vi "teleop3.vi"() -> ()   [LabVIEW 2012, in "Test.lvrbt"]
uses:
  Test.lvrbt
  <vilib>/NXT/Hardware/Plugins/Tetrix DC Motor/TetrixDCMotorAddress.ctl
  <vilib>/NXT/Block Support/NXT_OutputPort.ctl
  <vilib>/NXT/NXTIO Xnodes/NXTIONodeSubVIs/LEGOStopAllMotors.vi
  <vilib>/FTC/FTC Calculate Drive Power - Arcade Left.vi
  <vilib>/NXT/NXTIO Xnodes/NXTIONodeSubVIs/LEGOMoveAllMotors.vi
  <vilib>/FTC/FTC Interpret Motor Power From Right Y Axis.vi
  <vilib>/FTC/FTC Interpret Motor Power From Left Y Axis.vi
  <vilib>/NXT/NXTIO Xnodes/NXTIONodeSubVIs/TETRIX IO Move DC Motors.vi
  <vilib>/NXT/NXTIO Xnodes/NXTIONodeSubVIs/NXTMoveMotors.vi
  <vilib>/NXT/NXTIO Xnodes/NXTIONodeSubVIs/NXTStopMotors.vi
  <vilib>/NXT/NXTIO Xnodes/NXTIONodeSubVIs/TETRIX IO Stop DC Motors.vi
  <vilib>/NXT/NXTIO Xnodes/NXTIONodeSubVIs/TETRIX IO Check Battery.vi
  <vilib>/NXT/Hardware/Plugins/Open Port/OpenPortAddress.ctl
  <vilib>/NXT/Subs/LVHSConnector.ctl
  <vilib>/NXT/NXTIO Xnodes/NXTIOXNode/NXTIO.xnode
  <vilib>/NXT/NXTIO Xnodes/AddressXNode/NXTIOAddress.xnode
  <vilib>/NXT/LegoClasses/BrickReference/BrickReference.lvclass
panel:
  in  "Drive Power 3":i8=75 min=-100 max=100
  in  "Drive Power 2":i8=75 min=-100 max=100
  in  "Drive Power":i8=75 min=-100 max=100
  # "You may modify the code as needed for your robot. To test this program for an FTC match, open to the Remote Control Editor, select the \"Run Program\" tab, and choose \"Teleop\"."
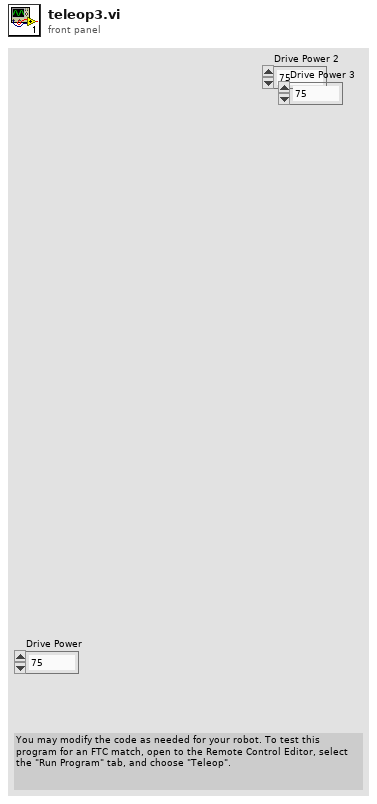
[diagram p1: front panel]
types:
  T1 = typedef "TetrixDCMotorAddress.ctl" = i32
  T2 = cluster{"TetrixDCMotor":T1, "TetrixDCMotor 2":T1}
  T3 = typedef "LVHSConnector.ctl" = refnum<class "BrickReference.lvclass">
  T4 = typedef "FTC ControllerState.ctl" = cluster{"Left X":i8, "Left Y":i8, "Right X":i8, "Right Y":i8, "Button Encoding 9-12":u8, "Button Encoding 1-8":u8, "POV":T5}
  T5 = typedef "FTC POVState.ctl" = i8
  T6 = typedef "FTC ButtonEventType.ctl" = enum16{"Pressed", "Released"}
  T7 = cluster{"Button ID":enum16{"None", "Button 1", "Button 2", "Button 3", "Button 4", "Button 5", "Button 6", "Button 7", "Button 8", "Button 9", "Button 10", "Button 11", "Button 12", "POV Up", "POV Up Right", "POV Right", "POV Down Right", "POV Down", "POV Down Left", "POV Left", "POV Up Left"}, "Event Type":T6}[]
  T8 = enum16{"None", "Button 1", "Button 2", "Button 3", "Button 4", "Button 5", "Button 6", "Button 7", "Button 8", "Button 9", "Button 10", "Button 11", "Button 12", "POV Up", "POV Up Right", "POV Right", "POV Down Right", "POV Down", "POV Down Left", "POV Left", "POV Up Left"}
  T9 = typedef "NXT_OutputPort.ctl" = u8
  T10 = typedef "FTC ButtonState.ctl" = cluster{"Button 1":bool, "Button 2":bool, "Button 3":bool, "Button 4":bool, "Button 5":bool, "Button 6":bool, "Button 7":bool, "Button 8":bool, "Button 9":bool, "Button 10":bool, "Button 11":bool, "Button 12":bool, "POV":T5}
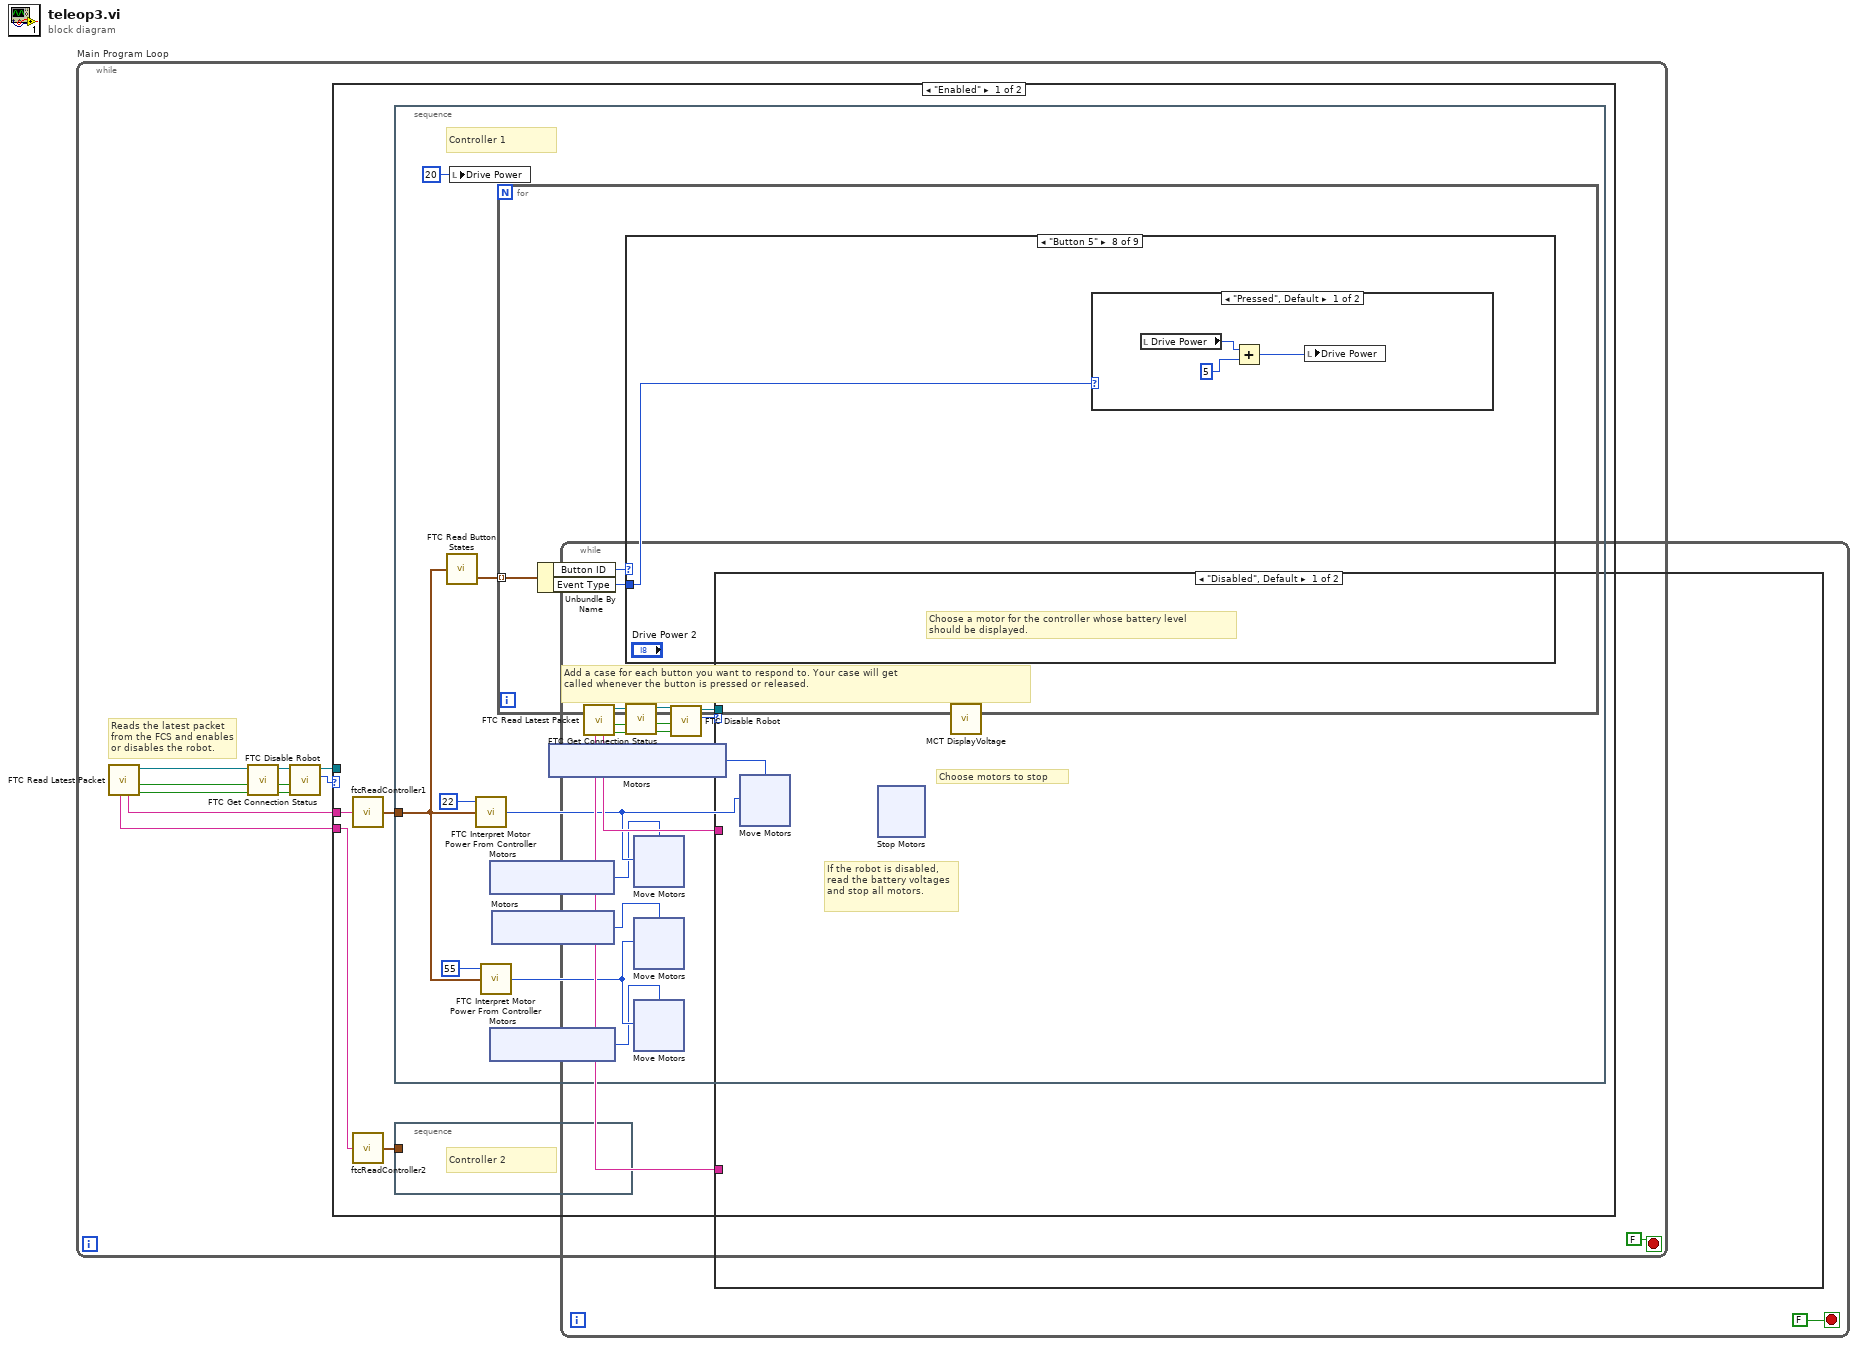
[diagram p0: block diagram]
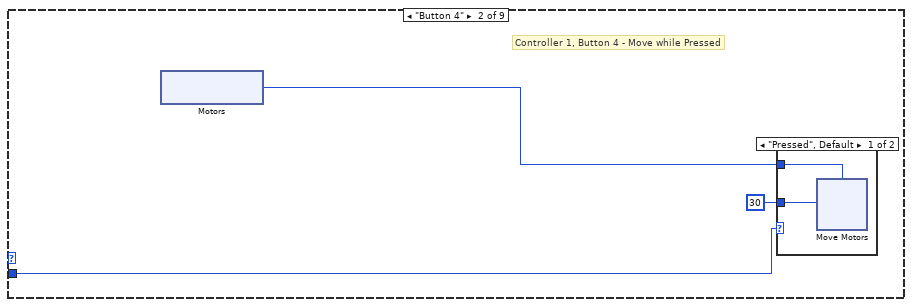
[diagram p3: hidden frame]
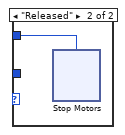
[diagram p4: hidden frame]
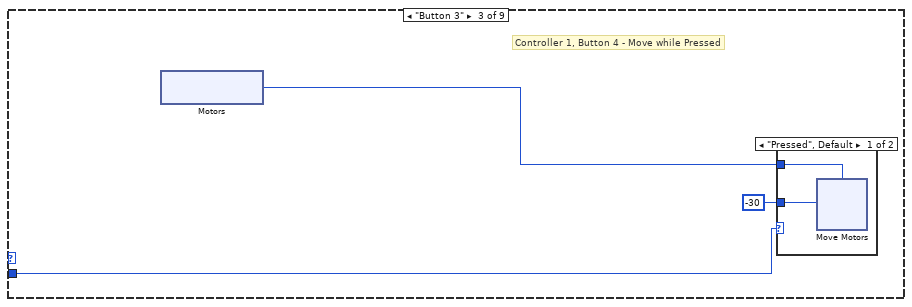
[diagram p5: hidden frame]
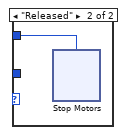
[diagram p6: hidden frame]
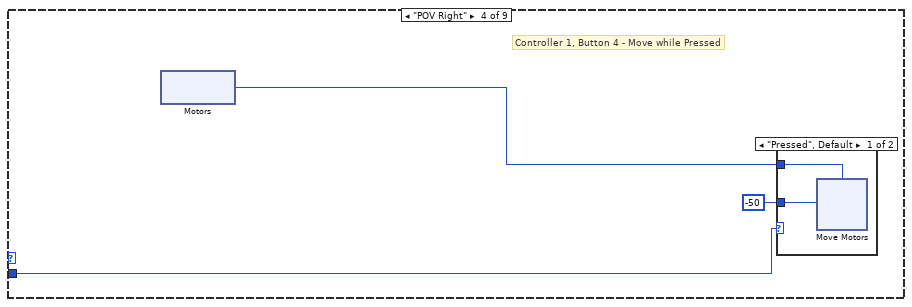
[diagram p7: hidden frame]
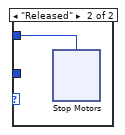
[diagram p8: hidden frame]
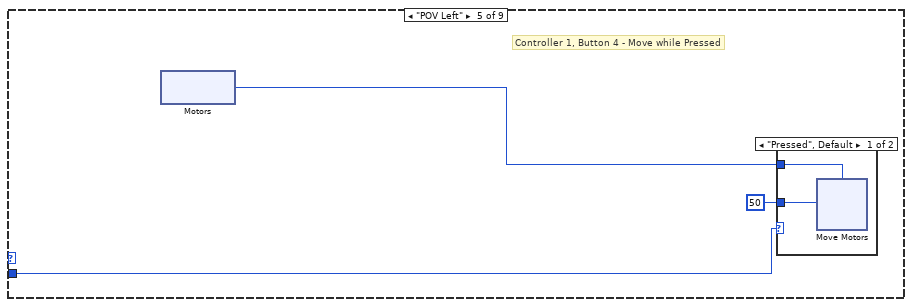
[diagram p9: hidden frame]
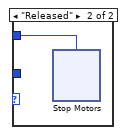
[diagram p10: hidden frame]
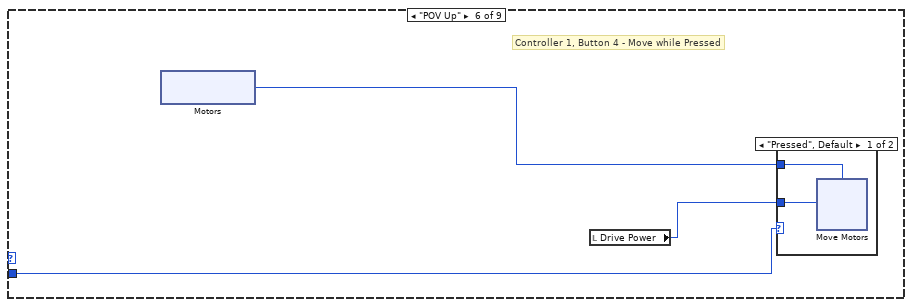
[diagram p11: hidden frame]
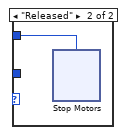
[diagram p12: hidden frame]
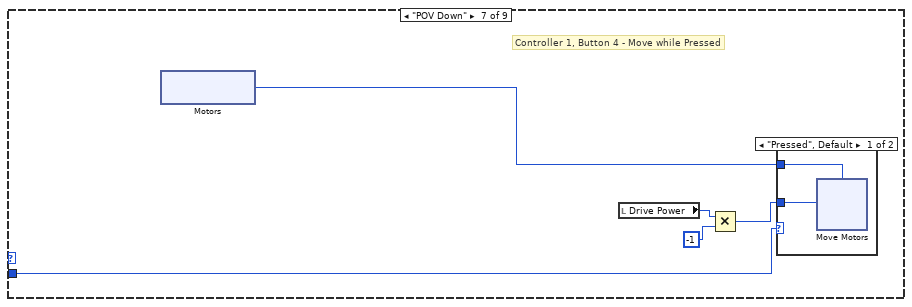
[diagram p13: hidden frame]
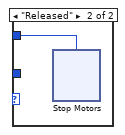
[diagram p14: hidden frame]
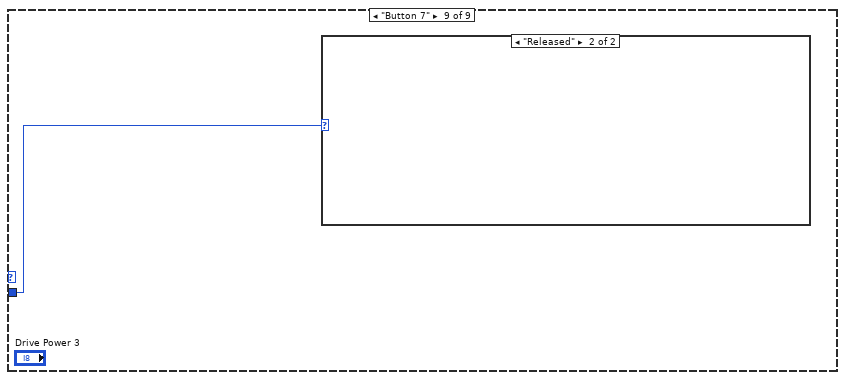
[diagram p16: hidden frame]
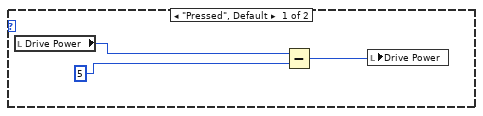
[diagram p17: hidden frame]
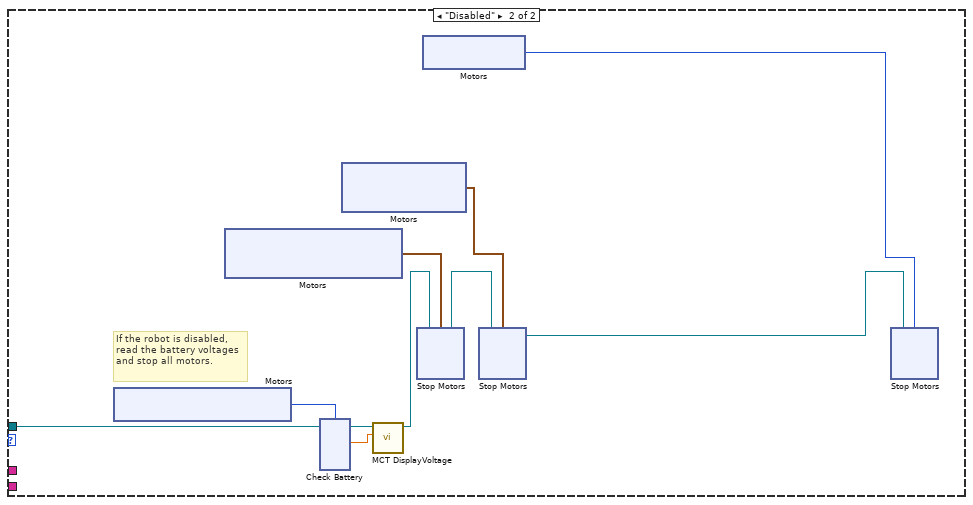
[diagram p18: hidden frame]
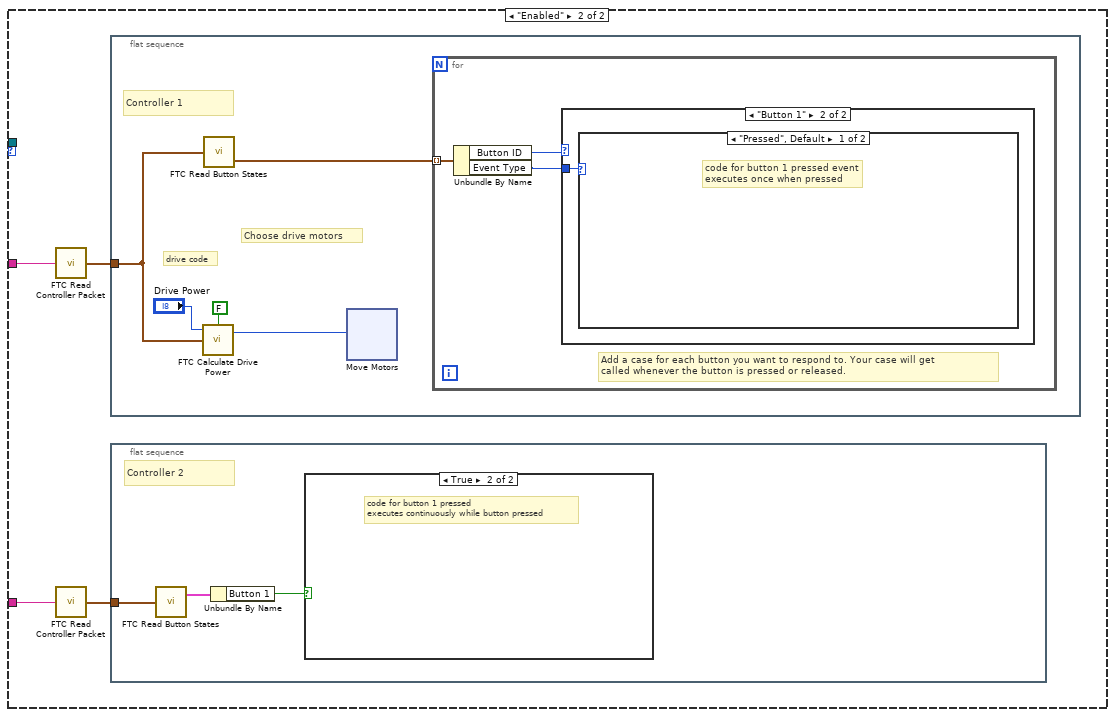
[diagram p19: hidden frame]
diagram:
  n1 = while "Main Program Loop" {
    stop <- FALSE stop-if-true
    # "Reads the latest packet\nfrom the FCS and enables\nor disables the robot."
    n2 = call <vilib>:"FTC Read Latest Packet.vi"() -> ("Packet Received?"=w8:bool, "Stopped?"=w5:bool, "NXT/EV3"=w7:T3, "Controller 1"=w10:string, "Controller 2"=w9:string)  [unwired: 6 in, 1 out]
    n3 = call <vilib>:"FTC Get Connection Status.vi"("Packet Received?"=w8, "Stopped?"=w5, "NXT/EV3"=w7) -> ("Online?"=w2:bool, "Stopped?"=w3:bool, "NXT/EV3"=w4:T3)  [unwired: 5 in]
    n4 = call <vilib>:"FTC Disable Robot.vi"("Online?"=w2, "Stopped?"=w3, "NXT/EV3"=w4) -> ("Enabled?"=w6:enum16{"Disabled", "Enabled"}, "NXT/EV3"=w1:T3)  [unwired: 3 in]
    n5 = case "disableCase" shown="\"Enabled\"" w6 {
      tunnel: w10 -> [w15 _]
      tunnel: w9 -> [w14 _]
      tunnel: w1 -> [_ w195]
      frame "Enabled" {
        n6 = call "ftcReadController1"("Packet"=w15) -> ("Controller State"=w13:T4)  [unwired: 4 in]
        n7 = call "ftcReadController2"("Packet"=w14) -> ("Controller State"=w12:T4)  [unwired: 4 in]
        n8 = stacked-sequence "controller1Actions" {
          tunnel: w13 -> [w25]
          frame #0 {
            # "Controller 1"
            n9 = call <vilib>:"FTC Read Button States.vi"("Controller State"=w25) -> ("Button Events"=w26:T7)  [unwired: 2 in, 1 out]
            n10 = local write "Drive Power"(i8 20 ("Drive Power")) -> ()
            n11 = call-poly <vilib>:"FTC Interpret Motor Power From Controller.vi"("Controller State"=w25, "Power Level (50)"=i8 22) -> ("Power"=w21:i8)  [unwired: 1 in]
            n12 = call-poly <vilib>:"FTC Interpret Motor Power From Controller.vi"("Controller State"=w25, "Power Level (50)"=i8 55) -> ("Power"=w20:i8)  [unwired: 1 in]
            n13 = xnode "Motors"() -> ("Motor"=w19:T1)
            n14 = xnode "Motors"() -> ("Motor"=w18:T1)
            n15 = xnode ("Motors")() -> ("Motor"=w17:T1)
            n16 = for "buttonAction" {
              tunnel: w26 -> [w59] mode=indexing
              # "Add a case for each button you want to respond to. Your case will get \ncalled whenever the button is pressed or released."
              n17 = Unbundle By Name(w59) -> ("Button ID"=w61:T8, "Event Type"=w60:T6)
              n18 = case "EventCase1" shown="\"Button 5\"" w61 {
                tunnel: w60 -> [_ w64 w83 w102 w121 w140 w161 w178 w182]
                frame Default {
                  # "No Action"
                }
                frame "Button 4" {
                  # "Controller 1, Button 4 - Move while Pressed"
                  n19 = xnode "Motors"() -> ("Motor"=w62:T9)
                  n20 = case shown="\"Pressed\", Default" w64 {
                    tunnel: 30 ("Power (75)") -> [w67 _]
                    tunnel: w62 -> [w66 w75]
                    frame "Pressed", Default {
                      n21 = xnode "Move Motors"("Power/Speed 1"=w67, "Motors"=w66) -> ()  [unwired: 1 in, 1 out]
                    }
                    frame "Released" {
                      n22 = xnode "Stop Motors"("Motors"=w75) -> ()  [unwired: 1 in, 1 out]
                    }
                  }
                }
                frame "Button 3" {
                  # "Controller 1, Button 4 - Move while Pressed"
                  n23 = xnode "Motors"() -> ("Motor"=w81:T9)
                  n24 = case shown="\"Pressed\", Default" w83 {
                    tunnel: -30 ("Power (75)") -> [w86 _]
                    tunnel: w81 -> [w85 w94]
                    frame "Pressed", Default {
                      n25 = xnode "Move Motors"("Power/Speed 1"=w86, "Motors"=w85) -> ()  [unwired: 1 in, 1 out]
                    }
                    frame "Released" {
                      n26 = xnode "Stop Motors"("Motors"=w94) -> ()  [unwired: 1 in, 1 out]
                    }
                  }
                }
                frame "POV Right" {
                  # "Controller 1, Button 4 - Move while Pressed"
                  n27 = xnode "Motors"() -> ("Motor"=w100:T1)
                  n28 = case shown="\"Pressed\", Default" w102 {
                    tunnel: -50 ("Power (75)") -> [w105 _]
                    tunnel: w100 -> [w104 w113]
                    frame "Pressed", Default {
                      n29 = xnode "Move Motors"("Power/Speed 1"=w105, "Motors"=w104) -> ()  [unwired: 1 in, 1 out]
                    }
                    frame "Released" {
                      n30 = xnode "Stop Motors"("Motors"=w113) -> ()  [unwired: 1 in, 1 out]
                    }
                  }
                }
                frame "POV Left" {
                  # "Controller 1, Button 4 - Move while Pressed"
                  n31 = xnode "Motors"() -> ("Motor"=w119:T1)
                  n32 = case shown="\"Pressed\", Default" w121 {
                    tunnel: 50 ("Power (75)") -> [w124 _]
                    tunnel: w119 -> [w123 w132]
                    frame "Pressed", Default {
                      n33 = xnode "Move Motors"("Power/Speed 1"=w124, "Motors"=w123) -> ()  [unwired: 1 in, 1 out]
                    }
                    frame "Released" {
                      n34 = xnode "Stop Motors"("Motors"=w132) -> ()  [unwired: 1 in, 1 out]
                    }
                  }
                }
                frame "POV Up" {
                  # "Controller 1, Button 4 - Move while Pressed"
                  n35 = xnode "Motors"() -> ("Motor"=w139:T1)
                  n36 = local read "Drive Power"() -> (w138:i8)
                  n37 = case shown="\"Pressed\", Default" w140 {
                    tunnel: w138 -> [w143 _]
                    tunnel: w139 -> [w142 w151]
                    frame "Pressed", Default {
                      n38 = xnode "Move Motors"("Power/Speed 1"=w143, "Motors"=w142) -> ()  [unwired: 1 in, 1 out]
                    }
                    frame "Released" {
                      n39 = xnode "Stop Motors"("Motors"=w151) -> ()  [unwired: 1 in, 1 out]
                    }
                  }
                }
                frame "POV Down" {
                  # "Controller 1, Button 4 - Move while Pressed"
                  n40 = xnode "Motors"() -> ("Motor"=w160:T1)
                  n41 = local read "Drive Power"() -> (w158:i8)
                  n42 = Multiply(x=w158, y=-1) -> (x*y=w157:i32)
                  n43 = case shown="\"Pressed\", Default" w161 {
                    tunnel: w157 -> [w164 _]
                    tunnel: w160 -> [w163 w172]
                    frame "Pressed", Default {
                      n44 = xnode "Move Motors"("Power/Speed 1"=w164, "Motors"=w163) -> ()  [unwired: 1 in, 1 out]
                    }
                    frame "Released" {
                      n45 = xnode "Stop Motors"("Motors"=w172) -> ()  [unwired: 1 in, 1 out]
                    }
                  }
                }
                frame "Button 5" {
                  n46 = case shown="\"Pressed\", Default" w178 {
                    frame "Pressed", Default {
                      n47 = local read "Drive Power"() -> (w180:i8)
                      n48 = Add(x=w180, y=5) -> (x+y=w179:i32)
                      n49 = local write "Drive Power"(w179) -> ()
                    }
                    frame "Released" {
                    }
                  }
                }
                frame "Button 7" {
                  n50 = case shown="\"Released\"" w182 {
                    frame "Pressed", Default {
                      n51 = local read "Drive Power"() -> (w184:i8)
                      n52 = Subtract(x=w184, y=5) -> (x-y=w183:i32)
                      n53 = local write "Drive Power"(w183) -> ()
                    }
                    frame "Released" {
                    }
                  }
                }
              }
            }
            n54 = xnode "Motors"() -> ("Motor"=w22:T1)
            n55 = xnode "Move Motors"("Power/Speed 1"=w21, "Motors"=w19) -> ()  [unwired: 1 in, 1 out]
            n56 = xnode ("Move Motors")("Power/Speed 1"=w20, "Motors"=w17) -> ()  [unwired: 1 in, 1 out]
            n57 = xnode "Move Motors"("Power/Speed 1"=w20, "Motors"=w18) -> ()  [unwired: 1 in, 1 out]
            n58 = xnode "Move Motors"("Power/Speed 1"=w21, "Motors"=w22) -> ()  [unwired: 1 in, 1 out]
          }
        }
        n59 = stacked-sequence "controller2Actions" {
          tunnel: w12 -> [_]
          frame #0 {
            # "Controller 2"
          }
        }
      }
      frame "Disabled" {
        # "If the robot is disabled, read the battery voltages and stop all motors."
        n60 = xnode ("Motors")() -> ("Motor"=w194:T1)
        n61 = xnode "Motors"() -> ("Motor"=w191:cluster{"TetrixDCMotor":T1, "TetrixDCMotor":T1})
        n62 = xnode ("Check Battery")("Motors"=w194, "NXT/EV3"=w195) -> ("Voltage 1"=w193:sgl, "NXT/EV3"=w192:T3)
        n63 = xnode "Motors"() -> ("Motor"=w189:cluster{"TetrixDCMotor":T1, "TetrixDCMotor":T1})
        n64 = call <vilib>:"MCT DisplayVoltage.vi"("Motor Voltage"=w193, "NXT/EV3"=w192) -> ("NXT/EV3"=w190:T3)  [unwired: 9 in]
        n65 = xnode "Stop Motors"("Motors"=w191, "NXT/EV3"=w190) -> ("NXT/EV3"=w188:T3)
        n66 = xnode "Motors"() -> ("Motor"=w187:T9)
        n67 = xnode "Stop Motors"("Motors"=w189, "NXT/EV3"=w188) -> ("NXT/EV3"=w186:T3)
        n68 = xnode "Stop Motors"("Motors"=w187, "NXT/EV3"=w186) -> ()  [unwired: 1 out]
      }
    }
  }
  n69 = while {
    stop <- FALSE stop-if-true
    n70 = call <vilib>:"FTC Read Latest Packet.vi"() -> ("Packet Received?"=w230:bool, "Stopped?"=w229:bool, "NXT/EV3"=w228:T3, "Controller 1"=w222:string, "Controller 2"=w221:string)  [unwired: 6 in, 1 out]
    n71 = call <vilib>:"FTC Get Connection Status.vi"("Packet Received?"=w230, "Stopped?"=w229, "NXT/EV3"=w228) -> ("Online?"=w227:bool, "Stopped?"=w226:bool, "NXT/EV3"=w225:T3)  [unwired: 5 in]
    n72 = call <vilib>:"FTC Disable Robot.vi"("Online?"=w227, "Stopped?"=w226, "NXT/EV3"=w225) -> ("Enabled?"=w224:enum16{"Disabled", "Enabled"}, "NXT/EV3"=w223:T3)  [unwired: 3 in]
    n73 = case shown="\"Disabled\", Default" w224 {
      tunnel: w223 -> [_ _]
      tunnel: w222 -> [_ w239]
      tunnel: w221 -> [_ w238]
      frame "Disabled", Default {
        # "Choose motors to stop"
        # "Choose a motor for the controller whose battery level \nshould be displayed."
        # "If the robot is disabled, read the battery voltages and stop all motors."
        n74 = xnode "Stop Motors"() -> ()  [unwired: 2 in, 1 out]
        n75 = call <vilib>:"MCT DisplayVoltage.vi"() -> ()  [unwired: 11 in, 1 out]
      }
      frame "Enabled" {
        n76 = call <vilib>:"FTC Read Controller Packet.vi"("Packet"=w239) -> ("Controller State"=w236:T4)  [unwired: 4 in]
        n77 = call <vilib>:"FTC Read Controller Packet.vi"("Packet"=w238) -> ("Controller State"=w237:T4)  [unwired: 4 in]
        n78 = flat-sequence {
          tunnel: w236 -> [w246]
          frame #0 {
            # "Choose drive motors"
            # "drive code"
            # "Controller 1"
            n79 = call-poly <vilib>:"FTC Calculate Drive Power.vi"("Reverse"=FALSE, "Controller State"=w246, "Power Level (50)"="Drive Power") -> ("Left Motor Power"=w243:i8)  [unwired: 1 in, 1 out]
            n80 = call <vilib>:"FTC Read Button States.vi"("Controller State"=w246) -> ("Button Events"=w247:T7)  [unwired: 2 in, 1 out]
            n81 = xnode "Move Motors"("Power/Speed 1"=w243) -> ()  [unwired: 2 in, 1 out]
            n82 = for {
              tunnel: w247 -> [w257] mode=indexing
              # "Add a case for each button you want to respond to. Your case will get \ncalled whenever the button is pressed or released."
              n83 = Unbundle By Name(w257) -> ("Button ID"=w256:T8, "Event Type"=w255:T6)
              n84 = case shown="\"Button 1\"" w256 {
                tunnel: w255 -> [_ w258]
                frame "None", Default {
                }
                frame "Button 1" {
                  n85 = case shown="\"Pressed\", Default" w258 {
                    frame "Pressed", Default {
                      # "code for button 1 pressed event\nexecutes once when pressed"
                    }
                    frame "Released" {
                    }
                  }
                }
              }
            }
          }
        }
        n86 = flat-sequence {
          tunnel: w237 -> [w242]
          frame #0 {
            # "Controller 2"
            n87 = call <vilib>:"FTC Read Button States.vi"("Controller State"=w242) -> ("Button States"=w241:T10)  [unwired: 2 in, 1 out]
            n88 = Unbundle By Name(w241) -> ("Button 1"=w240:bool)
            n89 = case shown="True" w240 {
              frame False {
              }
              frame True {
                # "code for button 1 pressed\nexecutes continuously while button pressed"
              }
            }
          }
        }
      }
    }
  }
